vi "[Dialog] - Help About.vi"(11 "Path":path=path "P:/~TecNOVA/~PROJECTS/2900.00 - S&C Calibration Console/builds/S&C Cal Console/S&C CAL Console.exe") -> ()   [LabVIEW 2015]
uses:
  TypeDefs_Utility/ENUM RB_Pos_Quadrant Position.ctl
  FP/FPClass/(FP)/DecFrame_FP/DecFrame_FP.lvclass
panel:
  out "FileDescription":string
  out "CompanyName":string
  out "Banner Text 2":string="Banner Text  ???????"
  out "LegalCopyright":string
  out "InternalName":string
  out "FileVersion":string
  out "ProductName":string
  out "Tab Control":enum32{"Client", "TECNOVA", "LabVIEW"}(tab)
  out "Banner Text":string="Picture Text???"
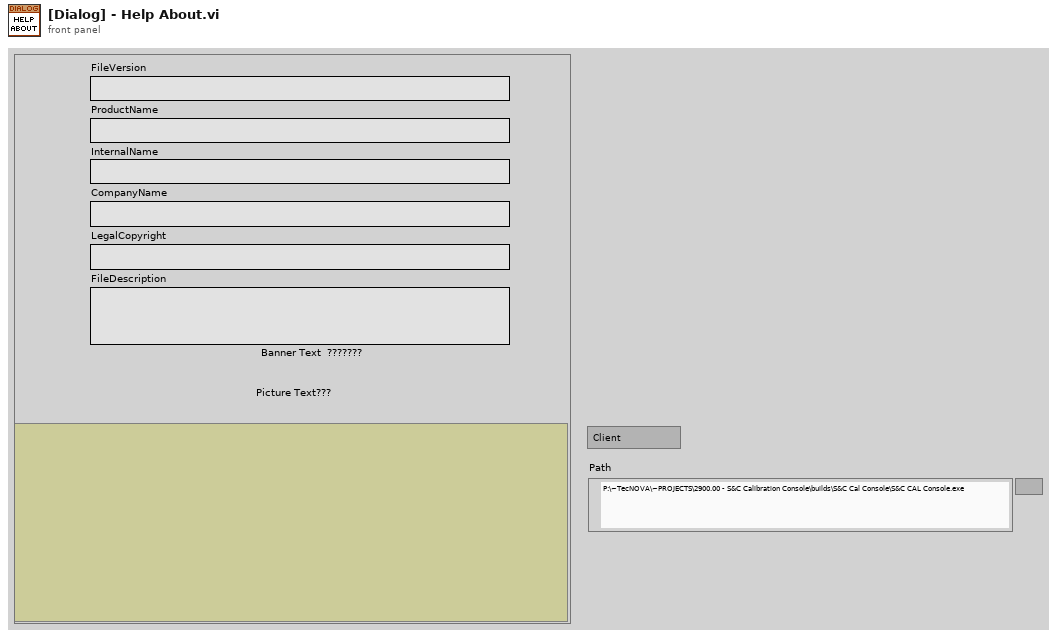
[diagram p1: front panel]
types:
  T1 = enum32{"Invalid", "Standard", "Closed", "Hidden", "Minimized", "Maximized"}
  T2 = typedef "ENUM RB_Pos_Quadrant Position.ctl" = enum32{"LFT-TOP", "MID-TOP", "RGT-TOP", "LFT-CTR", "MID-CTR", "RGT-CTR", "LFT-BOT", "MID-BOT", "RGT-BOT"}
  T3 = cluster{"Picture Text":string, "Display Time":i32, "Image":i32}[]
  T4 = typedef "FileVersionInformation.ctl" = cluster{"FileVersion":string, "ProductName":string, "InternalName":string, "CompanyName":string, "LegalCopyright":string, "FileDescription":string}
  T5 = cluster{"Picture Text":string, "Display Time":i32, "Image":i32}
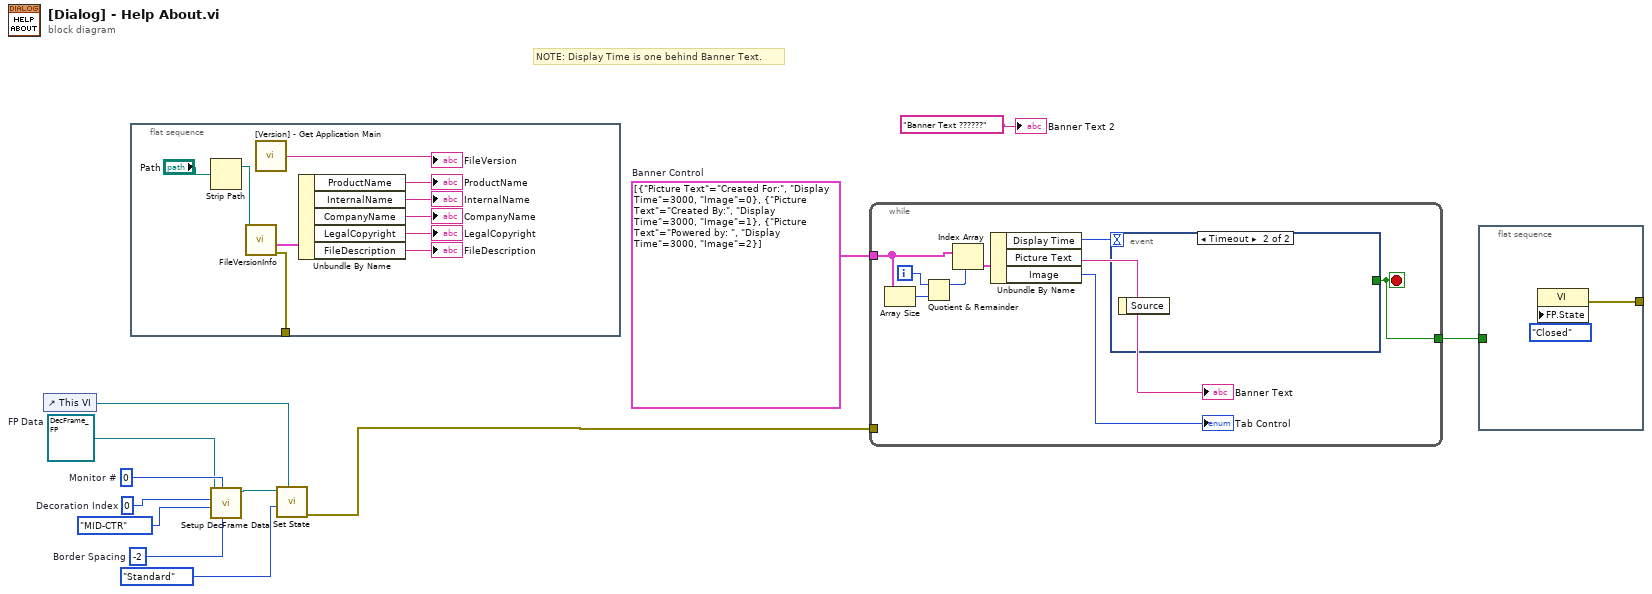
[diagram p0: block diagram]
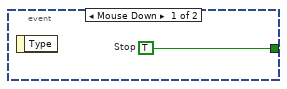
[diagram p2: hidden frame]
diagram:
  w1 = refnum<class "DecFrame_FP.lvclass"> refnum  # FP Data
  w9 = i16 -2  # Border Spacing
  w7 = 0  # Decoration Index
  w6 = u16 0  # Monitor #
  w12 = T3 [{"Picture Text"="Created For:", "Display Time"=3000, "Image"=0}, {"Picture Text"="Created By:", "Display Time"=3000, "Image"=1}, {"Picture Text"="Powered by: ", "Display Time"=3000, "Image"=2}]  # Banner Control
  # "NOTE: Display Time is one behind Banner Text."
  n1 = control-ref of="This VI"() -> (w3:refnum<vi>)
  n2 = flat-sequence {
    tunnel: [w14] -> _
    frame #0 {
      n3 = Strip Path(path="Path") -> (stripped path=w16:path)  [unwired: 1 out]
      n4 = call <vilib>:"FileVersionInfo.vi"("Application Path in"=w16) -> ("error out"=w14:errorcluster, "FileVersionInfo Out"=w15:T4)  [unwired: 7 in, 2 out]
      n5 = call "[Version] - Get Application Main.vi"() -> ("Version"=→"FileVersion":string)
      n6 = Unbundle By Name(w15) -> ("ProductName"=→"ProductName":string, "InternalName"=→"InternalName":string, "CompanyName"=→"CompanyName":string, "LegalCopyright"=→"LegalCopyright":string, "FileDescription"=→"FileDescription":string)
    }
  }
  n7 = call-dynamic "Setup DecFrame Data.vi"("Border Spacing"=w9, "Monitor #"=w6, "FPLocation"=ENUM_RB_Pos_Quadrant_Position."MID-CTR", "Decoration Index"=w7, "(FP)"=w1) -> ("(FP) Out"=w5:refnum<class "DecFrame_FP.lvclass">)  [unwired: 5 in, 1 out]
  n8 = call-dynamic "Set State.vi"("VI Ref"=w3, "State"=T1."Standard", "(FP)"=w5) -> ("Error Out"=w2:errorcluster)  [unwired: 6 in, 2 out]
  n9 = while {
    tunnel: w12 -> [w27]
    tunnel: w2 -> [_]
    tunnel: [w28] -> w11
    i -> [w30]
    stop <- w28 stop-if-true
    n10 = Array Size(array=w27) -> (size(s)=w31:i32)
    n11 = Quotient & Remainder(x=w30, y=w31) -> (x-y*floor(x/y)=w26:i32)  [unwired: 1 out]
    n12 = Index Array(array=w27, index=w26) -> (element=w29:T5)
    n13 = Unbundle By Name(w29) -> ("Display Time"=w23:i32, "Picture Text"=→"Banner Text":string, "Image"=→"Tab Control":i32)
    n14 = event shown="[1] Timeout" {
      selector: _ -> [_ _]
      dyn-events: _ -> [_ _]
      timeout: w23 -> [_ _]
      tunnel: [w32 _] -> w28
      event Mouse Down {
        w32 = TRUE  # Stop
        n15 = event-data() -> ()  [unwired: 1 in, 1 out]
      }
      event Timeout {
        n16 = event-data() -> ()  [unwired: 1 in, 1 out]
      }
    }
  }
  n17 = flat-sequence {
    tunnel: w11 -> [_]
    tunnel: [w33] -> _
    frame #0 {
      n18 = property class="VI"("FP.State"=T1."Closed" ("Front Panel Window:State")) -> (error out=w33:errorcluster)  [unwired: 2 in, 1 out]
    }
  }
  "Banner Text 2" <- "Banner Text ??????" ("Banner Text 2")
